vi "StateLED.vi"(0 "Master State In":T1(ring)) -> ()   [LabVIEW 2020]
doc: "This VI manages the apperance of the LEDs. The LED coloration and blink pattern report the robot mode and status. See project documentation for details."
uses:
  <vilib>/Rock Robotics/WPI/DriverStation/WPI_DriverStationRobotMode2.ctl
  GlobalPoseAndTargeting.vi
  GlobalArm.vi
  GlobalGripper.vi
  GlobalMiscellaneous.vi
  GlobalDriverStationData.vi
  GlobalDrivebase.vi
  GlobalAutonomous.vi
  <vilib>/vision/NI_Vision_Development_Module.lvlib
panel:
  in  "TOF Index":i32=11
  in  "TOF Insert":u32(colorbox)=65535
  in  "TOF Background":u32(colorbox)=16745472
  in  "TOF LED Length":i32=6
  in  "Human Player Signal":u32(colorbox)=65535
  in  "CONE":u32(colorbox)=16745472
  in  "CUBE":u32(colorbox)=8651007
  in  "Scoring":u32(colorbox)=65304
  in  "Balancing":u32(colorbox)=16711758
  in  "Human Control":u32(colorbox)=65280
  in  "Master Caution":u32(colorbox)=16736256
  in  "User Value Choice":u8(slide)=255 step=1 scale=0.0..255.0
  in  "User Saturation Choice":u8(slide)=255 step=1 scale=0.0..255.0
  in  "Pressure Insert":u32(colorbox)=91
  in  "Battery Insert":u32(colorbox)=65282
  in  "Pressure Background":u32(colorbox)=16711680
  in  "Battery Background":u32(colorbox)=16711680
  in  "Pressure LED Length":i32=6
  in  "Battery LED Length":i32=6
  in  "Battery Index":i32=4
  in  "Pressure Index":i32=4
  in  "Swerve 2 LED Index":i32
  in  "Swerve 3 LED Index":i32
  in  "Swerve 0 LED Index":i32=18
  in  "Swerve LED Length":i32=2
  in  "Swerve 1 LED Index":i32=18
  in  "Locate LED":bool
  in  "LED Index":i32
  out "User Blue":u8
  out "User Green":u8=255
  out "User Red":u8
  in  "Choose Hue":bool
  in  "User Hue Choice":u8(slide)=255 step=1 scale=0.0..255.0
  in  "Nominal":u32(colorbox)=65280
  in  "Master Alarm":u32(colorbox)=16711680
  in  "Robot Control":u32(colorbox)=16727040
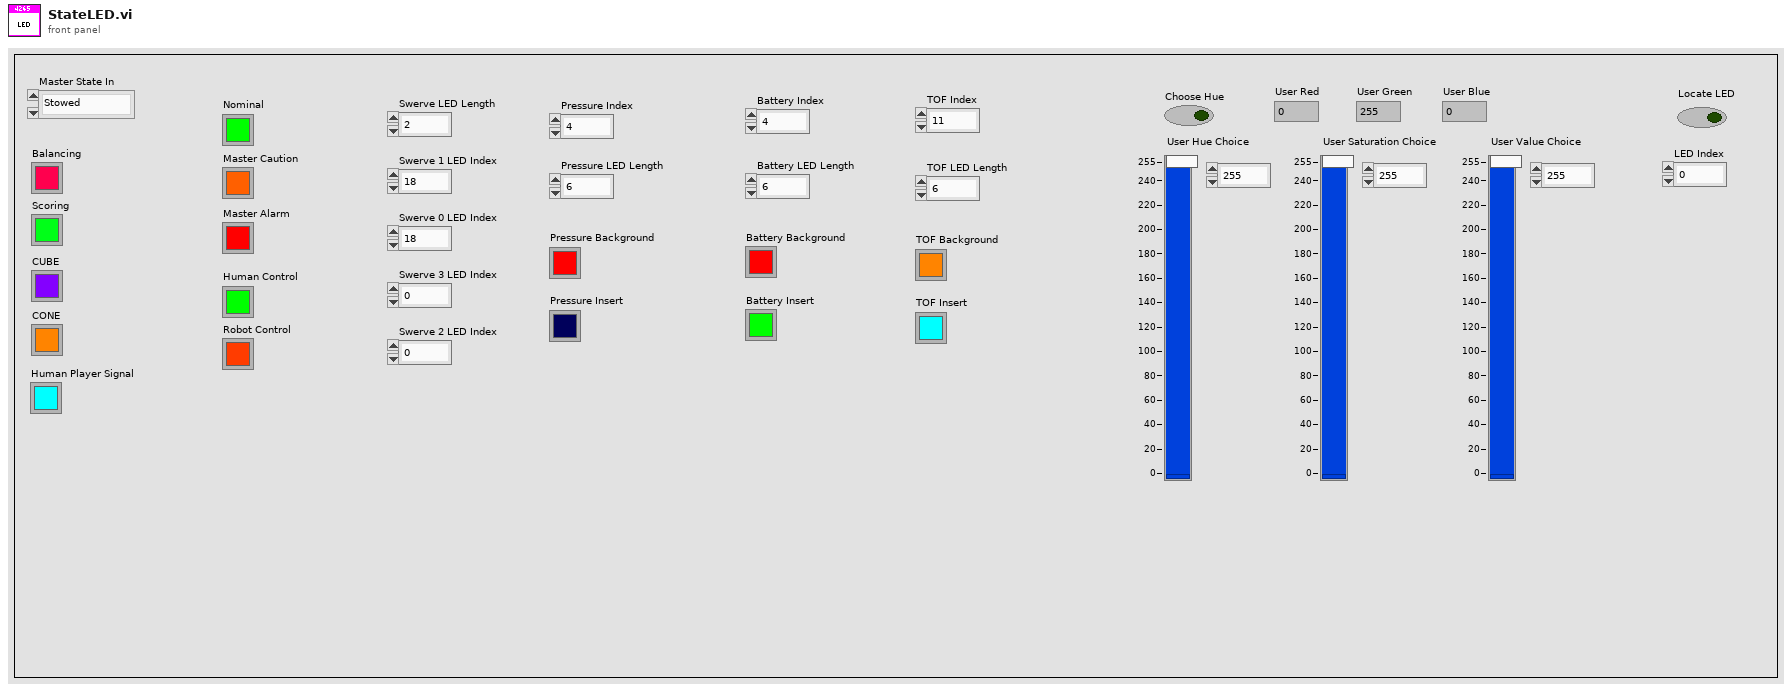
[diagram p1: front panel]
types:
  T1 = enum16{"Stowed", "Balancing", "Scoring", "Hoppering", "Ground", "Shelf"}
  T2 = enum16{"Normal", "Party Mode", "Choose Hue", "Debug", "Locate LED", "Distance Rainbow"}
  T3 = typedef "WPI_DriverStationRobotMode2.ctl" = enum16{"Autonomous Disabled", "Autonomous Enabled", "Teleop Disabled", "Teleop Enabled", "Disconnected", "Finish", "Test Disabled", "Test Enabled", "Emergency Stopped"}
  T4 = enum16{"Low Gear", "High Gear", "Transiting", "Unknown", "Force Low Gear"}
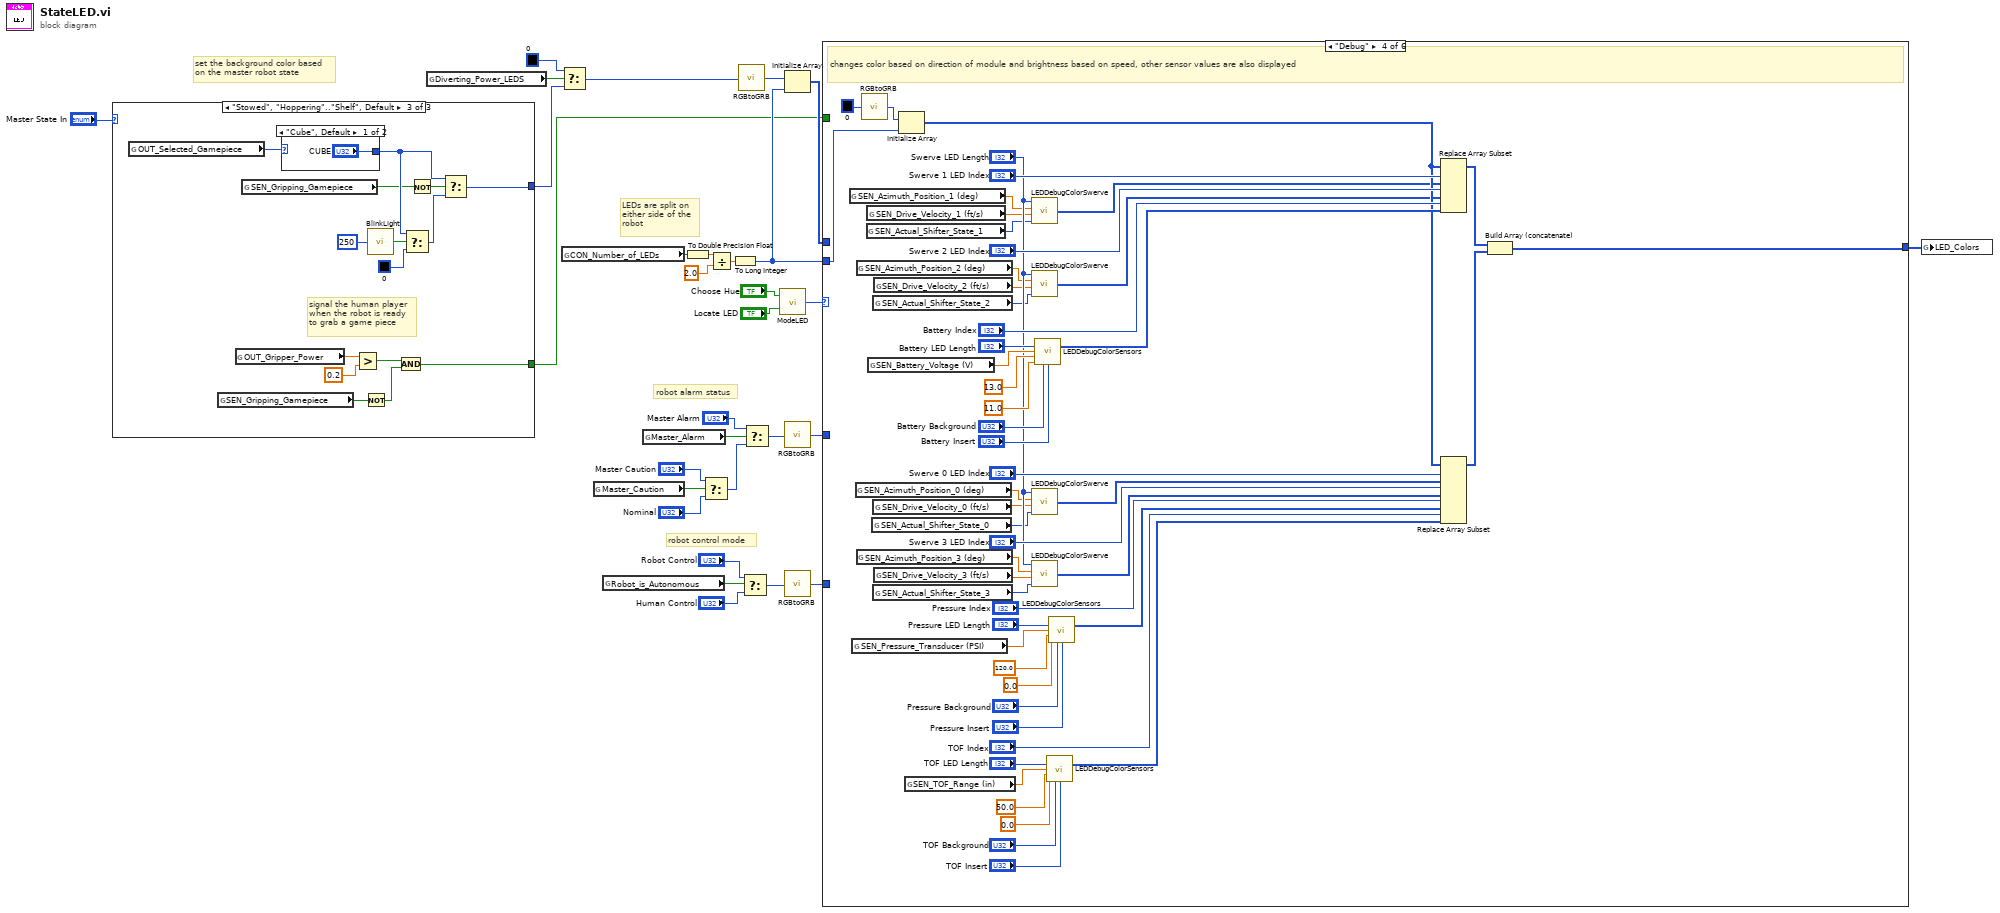
[diagram p0: block diagram]
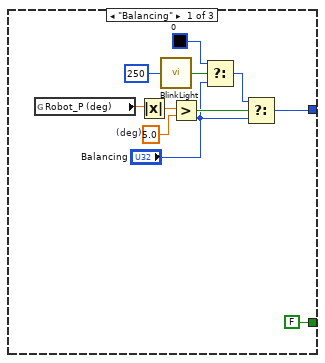
[diagram p2: hidden frame]
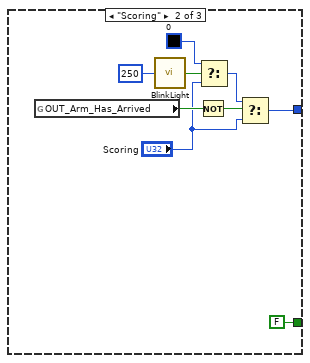
[diagram p3: hidden frame]
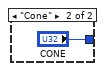
[diagram p4: hidden frame]
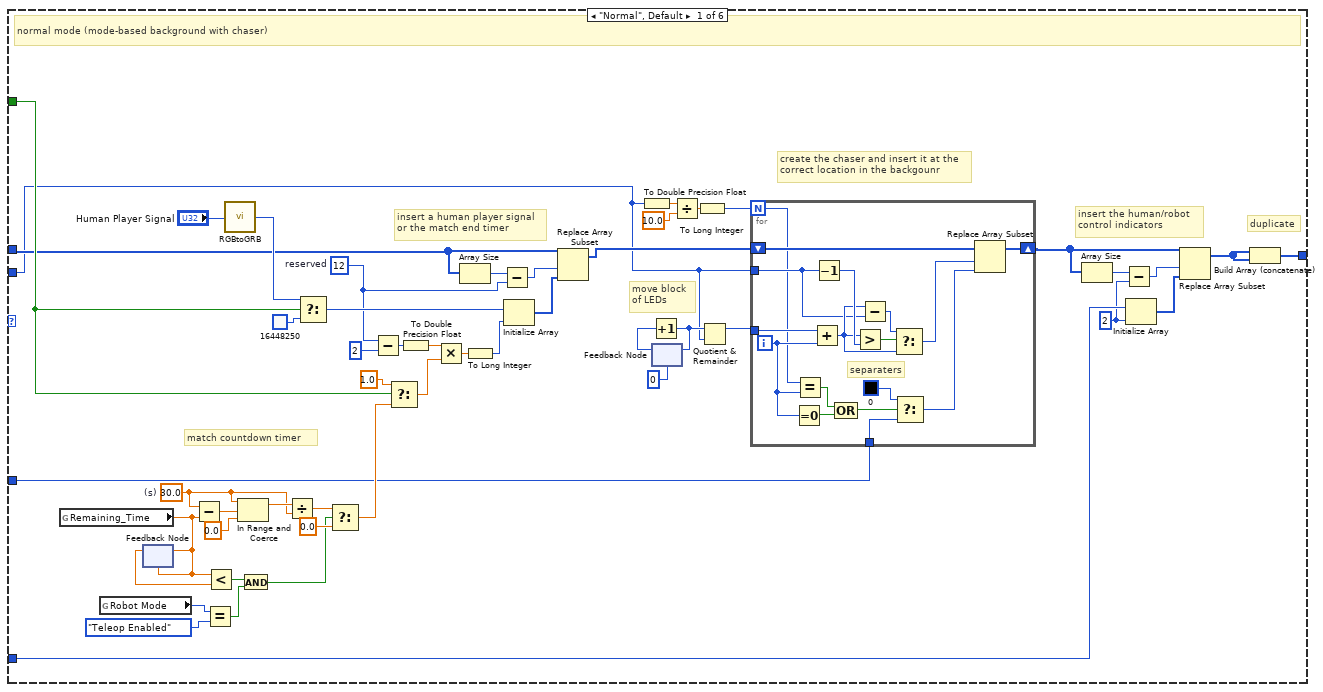
[diagram p5: hidden frame]
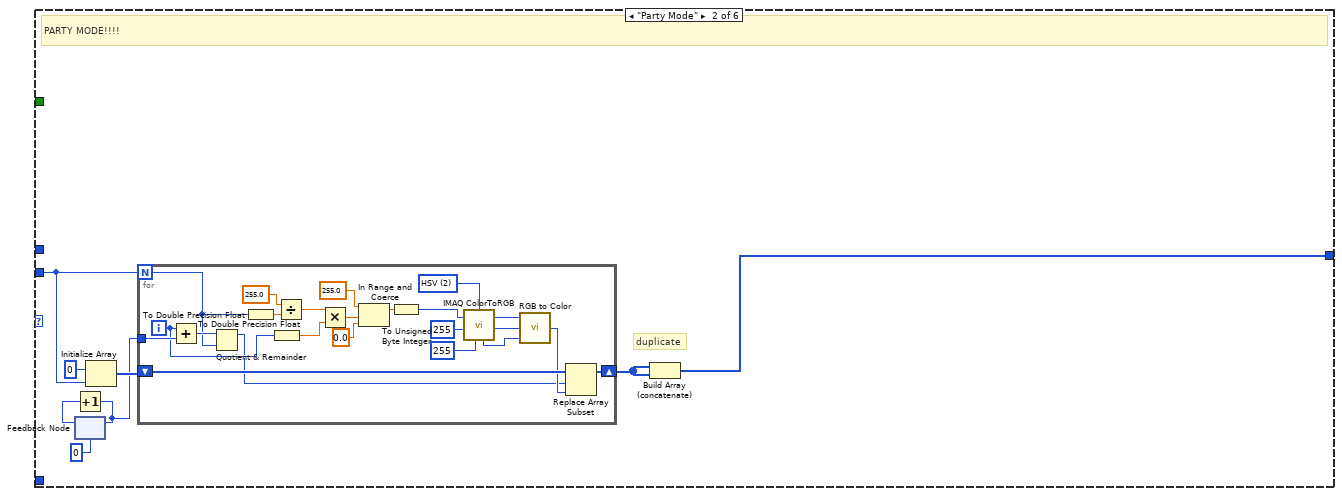
[diagram p6: hidden frame]
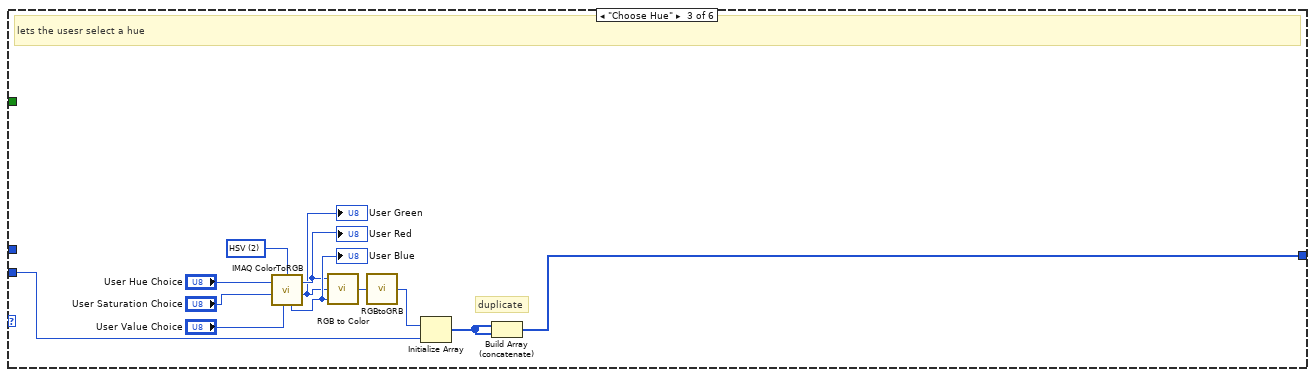
[diagram p7: hidden frame]
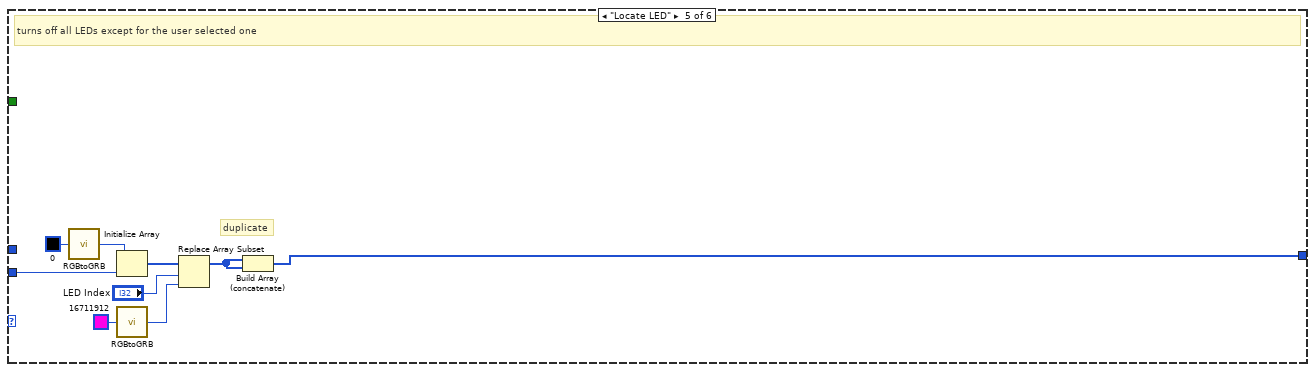
[diagram p8: hidden frame]
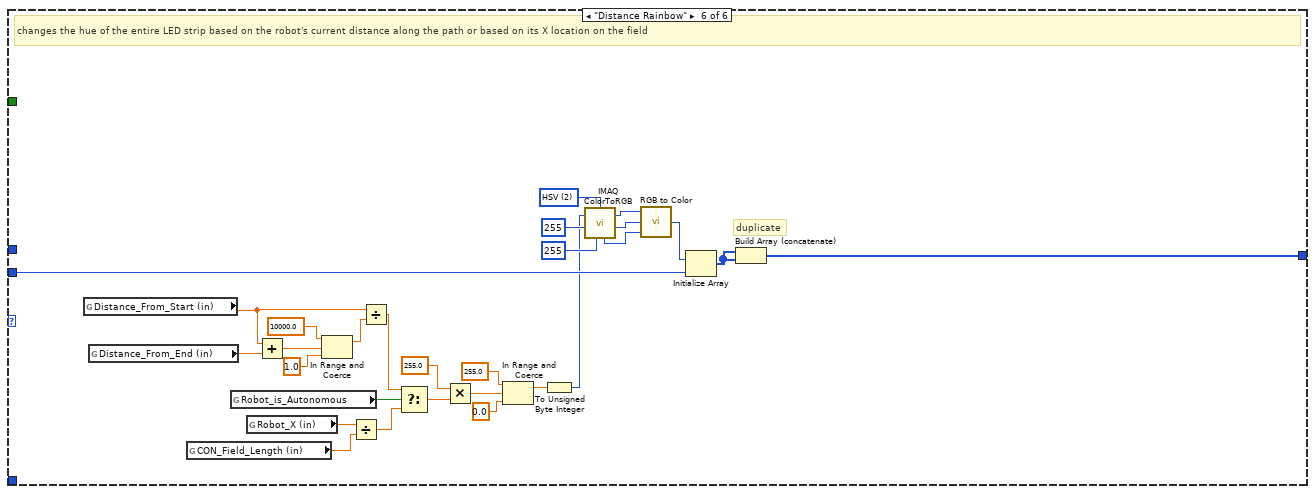
[diagram p9: hidden frame]
diagram:
  # "robot control mode"
  # "LEDs are split on\neither side of the \nrobot"
  # "robot alarm status"
  # "set the background color based\non the master robot state"
  n1 = case shown="\"Stowed\", \"Hoppering\"..\"Shelf\", Default" "Master State In" {
    tunnel: [w41 w46 w57] -> w2
    tunnel: [FALSE FALSE w51] -> w1
    frame "Balancing" {
      w38 = 5.0  # (deg)
      n2 = global read "GlobalPoseAndTargeting.vi" "Robot_P (deg)"() -> (w40:dbl)
      n3 = Absolute Value(x=w40) -> (abs(x)=w39:dbl)
      n4 = call "BlinkLight.vi"("Blink Interval (ms)"=u32 250) -> ("Blinked Output"=w35:bool)
      n5 = Greater?(x=w39, y=w38) -> (0:w37:bool)
      n6 = Select(t=u32 0 ("Color (RGB)"), s=w35, f="Balancing") -> (s? t:f=w32:u32)
      n7 = Select(t=w32, s=w37, f="Balancing") -> (s? t:f=w41:u32)
    }
    frame "Scoring" {
      n8 = global read "GlobalArm.vi" "OUT_Arm_Has_Arrived"() -> (w44:bool)
      n9 = call "BlinkLight.vi"("Blink Interval (ms)"=u32 250) -> ("Blinked Output"=w49:bool)
      n10 = Not(x=w44) -> (.not. x?=w45:bool)
      n11 = Select(t=u32 0 ("Color (RGB)"), s=w49, f="Scoring") -> (s? t:f=w47:u32)
      n12 = Select(t=w47, s=w45, f="Scoring") -> (s? t:f=w46:u32)
    }
    frame "Stowed", "Hoppering".."Shelf", Default {
      # "signal the human player\nwhen the robot is ready\nto grab a game piece"
      n13 = global read "GlobalArm.vi" "OUT_Selected_Gamepiece"() -> (w62:enum16{"Cube", "Cone"})
      n14 = global read "GlobalGripper.vi" "SEN_Gripping_Gamepiece"() -> (w55:bool)
      n15 = global read "GlobalGripper.vi" "OUT_Gripper_Power"() -> (w53:dbl)
      n16 = global read "GlobalGripper.vi" "SEN_Gripping_Gamepiece"() -> (w59:bool)
      n17 = case shown="\"Cube\", Default" w62 {
        tunnel: ["CUBE" "CONE"] -> w60
        frame "Cube", Default {
        }
        frame "Cone" {
        }
      }
      n18 = Greater?(x=w53, y=0.2) -> (0:w54:bool)
      n19 = Not(x=w55) -> (.not. x?=w56:bool)
      n20 = call "BlinkLight.vi"("Blink Interval (ms)"=u32 250) -> ("Blinked Output"=w64:bool)
      n21 = Compound Arithmetic op=AND(w54, w56) -> (w51:bool)
      n22 = Select(t=w60, s=w64, f=u32 0 ("Color (RGB)")) -> (s? t:f=w65:u32)
      n23 = Not(x=w59) -> (.not. x?=w58:bool)
      n24 = Select(t=w60, s=w58, f=w65) -> (s? t:f=w57:u32)
    }
  }
  n25 = global read "GlobalMiscellaneous.vi" "Diverting_Power_LEDS"() -> (w21:bool)
  n26 = Select(t=u32 0 ("Diverting Power"), s=w21, f=w2) -> (s? t:f=w4:u32)
  n27 = global read "GlobalMiscellaneous.vi" "CON_Number_of_LEDs"() -> (w10:u16)
  n28 = global read "GlobalMiscellaneous.vi" "Master_Caution"() -> (w14:bool)
  n29 = global read "GlobalDriverStationData.vi" "Robot_is_Autonomous"() -> (w19:bool)
  n30 = global read "GlobalMiscellaneous.vi" "Master_Alarm"() -> (w20:bool)
  n31 = To Double Precision Float(number=w10) -> (double precision float=w8:dbl)
  n32 = Select(t="Master Caution", s=w14, f="Nominal") -> (s? t:f=w13:u32)
  n33 = Divide(x=w8, y=2.0) -> (x/y=w9:dbl)
  n34 = To Long Integer(number=w9) -> (32bit integer=w22:i32)
  n35 = call "RGBtoGRB.vi"("Color (RGB)"=w4) -> ("Color (GRB)"=w30:u32)
  n36 = Select(t="Robot Control", s=w19, f="Human Control") -> (s? t:f=w18:u32)
  n37 = Select(t="Master Alarm", s=w20, f=w13) -> (s? t:f=w16:u32)
  n38 = call "ModeLED.vi"("Locate LED"="Locate LED", "Choose Hue"="Choose Hue") -> ("LED Mode"=w25:T2)
  n39 = Initialize Array(w30, w22) -> (w27:u32[])
  n40 = call "RGBtoGRB.vi"("Color (RGB)"=w16) -> ("Color (GRB)"=w15:u32)
  n41 = call "RGBtoGRB.vi"("Color (RGB)"=w18) -> ("Color (GRB)"=w26:u32)
  n42 = case shown="\"Debug\"" w25 {
    tunnel: w27 -> [w85 _ _ _ _ _]
    tunnel: [w111 w135 w166 w212 w230 w239] -> w3
    tunnel: w26 -> [w117 _ _ _ _ _]
    tunnel: w22 -> [w73 w138 w174 w228 w232 w259]
    tunnel: w15 -> [w76 _ _ _ _ _]
    tunnel: w1 -> [w100 _ _ _ _ _]
    frame "Normal", Default {
      w95 = 30.0  # (s)
      w87 = 12  # reserved
      w115 = 2 ("dimension size")
      # "create the chaser and insert it at the \ncorrect location in the backgounr"
      # "move block\nof LEDs"
      # "match countdown timer"
      # "insert a human player signal\nor the match end timer"
      # "duplicate"
      # "insert the human/robot\ncontrol indicators"
      # "normal mode (mode-based background with chaser)"
      n43 = global read "GlobalDriverStationData.vi" "Remaining_Time"() -> (w71:dbl)
      n44 = global read "GlobalDriverStationData.vi" "Robot Mode"() -> (w90:T3)
      n45 = feedback-in #1(w71) -> ()
      n46 = feedback #1(w71) -> (w72:dbl)
      n47 = Subtract(x=w95, y=w71) -> (x-y=w96:dbl)
      n48 = Equal?(x=w90, y=WPI_DriverStationRobotMode2."Teleop Enabled") -> (x = y?=w68:bool)
      n49 = Less?(x=w71, y=w72) -> (x < y?=w70:bool)
      n50 = call "RGBtoGRB.vi"("Color (RGB)"="Human Player Signal") -> ("Color (GRB)"=w101:u32)
      n51 = In Range and Coerce(upper limit=w95, x=w96, lower limit=0.0) -> (coerced(x)=w97:dbl)  [unwired: 1 out]
      n52 = And(x=w70, y=w68) -> (x .and. y?=w69:bool)
      n53 = Divide(x=w97, y=w95) -> (x/y=w94:dbl)
      n54 = Select(t=w101, s=w100, f=u32 16448250 ("Color")) -> (s? t:f=w99:u32)
      n55 = Select(t=w94, s=w69, f=0.0) -> (s? t:f=w92:dbl)
      n56 = Subtract(x=w87, y=2) -> (x-y=w88:i32)
      n57 = Select(t=1.0, s=w100, f=w92) -> (s? t:f=w102:dbl)
      n58 = To Double Precision Float(number=w88) -> (double precision float=w106:dbl)
      n59 = Multiply(x=w106, y=w102) -> (x*y=w105:dbl)
      n60 = Array Size(array=w85) -> (size(s)=w109:i32)
      n61 = To Long Integer(number=w105) -> (32bit integer=w104:i32)
      n62 = Subtract(x=w109, y=w87) -> (x-y=w108:i32)
      n63 = Initialize Array(w99, w104) -> (w107:u32[])
      n64 = Replace Array Subset(array=w85, new element=w107, index=w108) -> (w74:u32[])
      n65 = To Double Precision Float(number=w73) -> (double precision float=w84:dbl)
      n66 = feedback #2(0) -> (w79:i32)
      n67 = Increment(x=w79) -> (x+1=w78:i32)
      n68 = feedback-in #2(w78) -> ()
      n69 = Divide(x=w84, y=10.0) -> (x/y=w83:dbl)
      n70 = To Long Integer(number=w83) -> (32bit integer=w75:i32)
      n71 = Quotient & Remainder(x=w78, y=w73) -> (x-y*floor(x/y)=w81:i32)  [unwired: 1 out]
      n72 = for {
        N: w75 -> [w118]
        tunnel: w81 -> [w134]
        tunnel: w73 -> [w127]
        shift-right: [w129] -> w77
        shift-left: w74 -> [w130]
        tunnel: w76 -> [w124]
        i -> [w119]
        # "separaters"
        n73 = Equal To 0?(x=w119) -> (x = 0?=w122:bool)
        n74 = Equal?(x=w118, y=w119) -> (x = y?=w120:bool)
        n75 = Add(x=w134, y=w119) -> (x+y=w128:i32)
        n76 = Decrement(x=w127) -> (x-1=w133:i32)
        n77 = Compound Arithmetic op=OR(w120, w122) -> (w121:bool)
        n78 = Greater?(x=w128, y=w133) -> (0:w132:bool)
        n79 = Subtract(x=w128, y=w127) -> (x-y=w126:i32)
        n80 = Select(t=w126, s=w132, f=w128) -> (s? t:f=w131:i32)
        n81 = Select(t=u32 0 ("Color (RGB)"), s=w121, f=w124) -> (s? t:f=w123:u32)
        n82 = Replace Array Subset(array=w130, new element=w123, index=w131) -> (w129:u32[])
      }
      n83 = Array Size(array=w77) -> (size(s)=w116:i32)
      n84 = Subtract(x=w116, y=w115) -> (x-y=w114:i32)
      n85 = Initialize Array(w117, w115) -> (w113:u32[])
      n86 = Replace Array Subset(array=w77, new element=w113, index=w114) -> (w112:u32[])
      n87 = Build Array (concatenate)(w112, w112) -> (w111:u32[])
    }
    frame "Party Mode" {
      # "duplicate"
      # "PARTY MODE!!!!"
      n88 = feedback #3(0) -> (w140:i32)
      n89 = Increment(x=w140) -> (x+1=w137:i32)
      n90 = feedback-in #3(w137) -> ()
      n91 = Initialize Array(u32 0 ("element"), w138) -> (w141:u32[])
      n92 = for {
        N: w138 -> [w145]
        shift-right: [w153] -> w136
        shift-left: w141 -> [w154]
        tunnel: w137 -> [w147]
        i -> [w144]
        w163 = u16 2 items=["RGB", "HSL", "HSV", "HSI"] ("Color Mode")
        n93 = Add(x=w144, y=w147) -> (x+y=w146:i32)
        n94 = Quotient & Remainder(x=w146, y=w145) -> (x-y*floor(x/y)=w143:i32)  [unwired: 1 out]
        n95 = To Double Precision Float(number=w145) -> (double precision float=w162:dbl)
        n96 = To Double Precision Float(number=w144) -> (double precision float=w159:dbl)
        n97 = Divide(x=255.0, y=w162) -> (x/y=w160:dbl)
        n98 = Multiply(x=w160, y=w159) -> (x*y=w158:dbl)
        n99 = In Range and Coerce(upper limit=255.0, x=w158, lower limit=0.0) -> (coerced(x)=w155:dbl)  [unwired: 1 out]
        n100 = To Unsigned Byte Integer(number=w155) -> (unsigned 8bit integer=w148:u8)
        n101 = call "IMAQ ColorToRGB"("Green or Sat value"=u8 255, "Blue or Luma or Val or Inten value"=u8 255, "Red or Hue value"=w148, "Color Mode"=w163) -> ("Blue value"=w149:u8, "Green value"=w150:u8, "Red value"=w151:u8)  [unwired: 1 in, 1 out]
        n102 = call <vilib>:"RGB to Color.vi"("B"=w149, "G"=w150, "R"=w151) -> ("Color"=w152:u32)
        n103 = Replace Array Subset(array=w154, new element=w152, index=w143) -> (w153:u32[])
      }
      n104 = Build Array (concatenate)(w136, w136) -> (w135:u32[])
    }
    frame "Choose Hue" {
      w175 = u16 2 items=["RGB", "HSL", "HSV", "HSI"] ("Color Mode")
      # "duplicate"
      # "lets the usesr select a hue"
      n105 = call "IMAQ ColorToRGB"("Green or Sat value"="User Saturation Choice", "Blue or Luma or Val or Inten value"="User Value Choice", "Red or Hue value"="User Hue Choice", "Color Mode"=w175) -> ("Blue value"=w176:u8, "Green value"=w170:u8, "Red value"=w171:u8)  [unwired: 1 in, 1 out]
      "User Red" <- w171
      "User Green" <- w170
      "User Blue" <- w176
      n106 = call <vilib>:"RGB to Color.vi"("B"=w176, "G"=w170, "R"=w171) -> ("Color"=w169:u32)
      n107 = call "RGBtoGRB.vi"("Color (RGB)"=w169) -> ("Color (GRB)"=w168:u32)
      n108 = Initialize Array(w168, w174) -> (w167:u32[])
      n109 = Build Array (concatenate)(w167, w167) -> (w166:u32[])
    }
    frame "Debug" {
      # "changes color based on direction of module and brightness based on speed, other sensor values are also displayed"
      n110 = global read "GlobalDrivebase.vi" "SEN_Azimuth_Position_1 (deg)"() -> (w197:dbl)
      n111 = global read "GlobalMiscellaneous.vi" "SEN_Pressure_Transducer (PSI)"() -> (w217:dbl)
      n112 = global read "GlobalDrivebase.vi" "SEN_Azimuth_Position_0 (deg)"() -> (w191:dbl)
      n113 = global read "GlobalDrivebase.vi" "SEN_Azimuth_Position_2 (deg)"() -> (w193:dbl)
      n114 = global read "GlobalDrivebase.vi" "SEN_Azimuth_Position_3 (deg)"() -> (w188:dbl)
      n115 = call "RGBtoGRB.vi"("Color (RGB)"=u32 0) -> ("Color (GRB)"=w214:u32)
      n116 = global read "GlobalDrivebase.vi" "SEN_Actual_Shifter_State_1"() -> (w195:T4)
      n117 = global read "GlobalDrivebase.vi" "SEN_Drive_Velocity_1 (ft/s)"() -> (w196:dbl)
      n118 = global read "GlobalMiscellaneous.vi" "SEN_Battery_Voltage (V)"() -> (w216:dbl)
      n119 = global read "GlobalDrivebase.vi" "SEN_Actual_Shifter_State_0"() -> (w189:T4)
      n120 = global read "GlobalDrivebase.vi" "SEN_Actual_Shifter_State_2"() -> (w192:T4)
      n121 = global read "GlobalDrivebase.vi" "SEN_Drive_Velocity_0 (ft/s)"() -> (w190:dbl)
      n122 = global read "GlobalDrivebase.vi" "SEN_Actual_Shifter_State_3"() -> (w186:T4)
      n123 = global read "GlobalDrivebase.vi" "SEN_Drive_Velocity_2 (ft/s)"() -> (w194:dbl)
      n124 = global read "GlobalDrivebase.vi" "SEN_Drive_Velocity_3 (ft/s)"() -> (w187:dbl)
      n125 = Initialize Array(w214, w228) -> (w208:u32[])
      n126 = global read "GlobalMiscellaneous.vi" "SEN_TOF_Range (in)"() -> (w180:dbl)
      n127 = call "LEDDebugColorSwerve.vi"("Shifter State"=w195, "Drive Velocity (ft/s)"=w196, "Azimuth Angle (deg [-180,180])"=w197, "Swerve LED Length"="Swerve LED Length") -> ("Color Array"=w202:u32[])
      n128 = call "LEDDebugColorSwerve.vi"("Shifter State"=w192, "Drive Velocity (ft/s)"=w194, "Azimuth Angle (deg [-180,180])"=w193, "Swerve LED Length"="Swerve LED Length") -> ("Color Array"=w201:u32[])
      n129 = call "LEDDebugColorSwerve.vi"("Shifter State"=w189, "Drive Velocity (ft/s)"=w190, "Azimuth Angle (deg [-180,180])"=w191, "Swerve LED Length"="Swerve LED Length") -> ("Color Array"=w200:u32[])
      n130 = call "LEDDebugColorSwerve.vi"("Shifter State"=w186, "Drive Velocity (ft/s)"=w187, "Azimuth Angle (deg [-180,180])"=w188, "Swerve LED Length"="Swerve LED Length") -> ("Color Array"=w199:u32[])
      n131 = call "LEDDebugColorSensors.vi"("LED Length"="Battery LED Length", "Value"=w216, "Max"=13.0, "Min"=11.0, "Background Color"="Battery Background", "Color to Insert"="Battery Insert") -> ("Output Color Array"=w209:u32[])  [unwired: 9 in]
      n132 = call "LEDDebugColorSensors.vi"("LED Length"="TOF LED Length", "Value"=w180, "Max"=50.0, "Min"=0.0, "Background Color"="TOF Background", "Color to Insert"="TOF Insert") -> ("Output Color Array"=w179:u32[])  [unwired: 9 in]
      n133 = call "LEDDebugColorSensors.vi"("LED Length"="Pressure LED Length", "Value"=w217, "Max"=120.0, "Min"=0.0, "Background Color"="Pressure Background", "Color to Insert"="Pressure Insert") -> ("Output Color Array"=w203:u32[])  [unwired: 9 in]
      n134 = Replace Array Subset(array=w208, new element #1=w202, index #1="Swerve 1 LED Index", new element #2=w201, index #2="Swerve 2 LED Index", new element #3=w209, index #3="Battery Index") -> (w213:u32[])
      n135 = Replace Array Subset(array=w208, new element #1=w200, index #1="Swerve 0 LED Index", new element #2=w199, index #2="Swerve 3 LED Index", new element #3=w203, index #3="Pressure Index", new element #4=w179, index #4="TOF Index") -> (w207:u32[])
      n136 = Build Array (concatenate)(w213, w207) -> (w212:u32[])
    }
    frame "Locate LED" {
      # "duplicate"
      # "turns off all LEDs except for the user selected one"
      n137 = call "RGBtoGRB.vi"("Color (RGB)"=u32 0) -> ("Color (GRB)"=w237:u32)
      n138 = Initialize Array(w237, w232) -> (w236:u32[])
      n139 = call "RGBtoGRB.vi"("Color (RGB)"=u32 16711912) -> ("Color (GRB)"=w234:u32)
      n140 = Replace Array Subset(array=w236, new element=w234, index="LED Index") -> (w231:u32[])
      n141 = Build Array (concatenate)(w231, w231) -> (w230:u32[])
    }
    frame "Distance Rainbow" {
      w263 = u16 2 items=["RGB", "HSL", "HSV", "HSI"] ("Color Mode")
      # "duplicate"
      # "changes the hue of the entire LED strip based on the robot's current distance along the path or based on its X location on the field"
      n142 = global read "GlobalAutonomous.vi" "Distance_From_Start (in)"() -> (w253:dbl)
      n143 = global read "GlobalAutonomous.vi" "Distance_From_End (in)"() -> (w258:dbl)
      n144 = global read "GlobalPoseAndTargeting.vi" "CON_Field_Length (in)"() -> (w241:dbl)
      n145 = global read "GlobalDriverStationData.vi" "Robot_is_Autonomous"() -> (w242:bool)
      n146 = global read "GlobalPoseAndTargeting.vi" "Robot_X (in)"() -> (w248:dbl)
      n147 = Add(x=w253, y=w258) -> (x+y=w257:dbl)
      n148 = In Range and Coerce(upper limit=10000.0 ("x"), x=w257, lower limit=1.0) -> (coerced(x)=w254:dbl)  [unwired: 1 out]
      n149 = Divide(x=w248, y=w241) -> (x/y=w243:dbl)
      n150 = Divide(x=w253, y=w254) -> (x/y=w252:dbl)
      n151 = Select(t=w252, s=w242, f=w243) -> (s? t:f=w251:dbl)
      n152 = Multiply(x=255.0, y=w251) -> (x*y=w245:dbl)
      n153 = In Range and Coerce(upper limit=255.0 ("x"), x=w245, lower limit=0.0) -> (coerced(x)=w244:dbl)  [unwired: 1 out]
      n154 = To Unsigned Byte Integer(number=w244) -> (unsigned 8bit integer=w249:u8)
      n155 = call "IMAQ ColorToRGB"("Green or Sat value"=u8 255 ("User Saturation Choice 2"), "Blue or Luma or Val or Inten value"=u8 255 ("User Value Choice 2"), "Red or Hue value"=w249, "Color Mode"=w263) -> ("Blue value"=w266:u8, "Green value"=w265:u8, "Red value"=w264:u8)  [unwired: 1 in, 1 out]
      n156 = call <vilib>:"RGB to Color.vi"("B"=w266, "G"=w265, "R"=w264) -> ("Color"=w262:u32)
      n157 = Initialize Array(w262, w259) -> (w240:u32[])
      n158 = Build Array (concatenate)(w240, w240) -> (w239:u32[])
    }
  }
  n159 = global write "GlobalMiscellaneous.vi" "LED_Colors"(w3) -> ()
